vi "Rename LVClass_rcf.vi"(7 "App reference":refnum<vi>, 8 "error in (no error)":errorcluster, 10 "New Class Name":string, 11 "LVClass Path":path) -> (0 "error out":errorcluster, 3 "Updated LVClass Path":path)   [LabVIEW 2009]
uses:
  <userlib>/_OpenG.lib/file/file.llb/Strip Path Extension - String__ogtk.vi
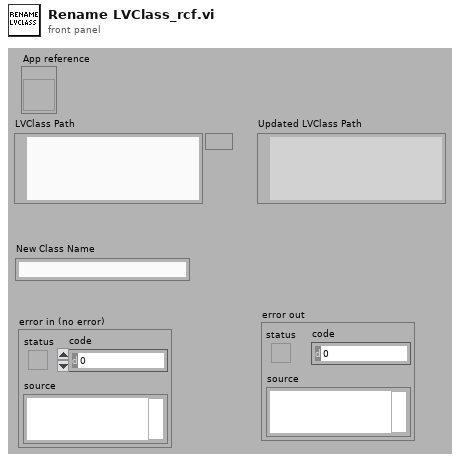
[diagram p1: front panel]
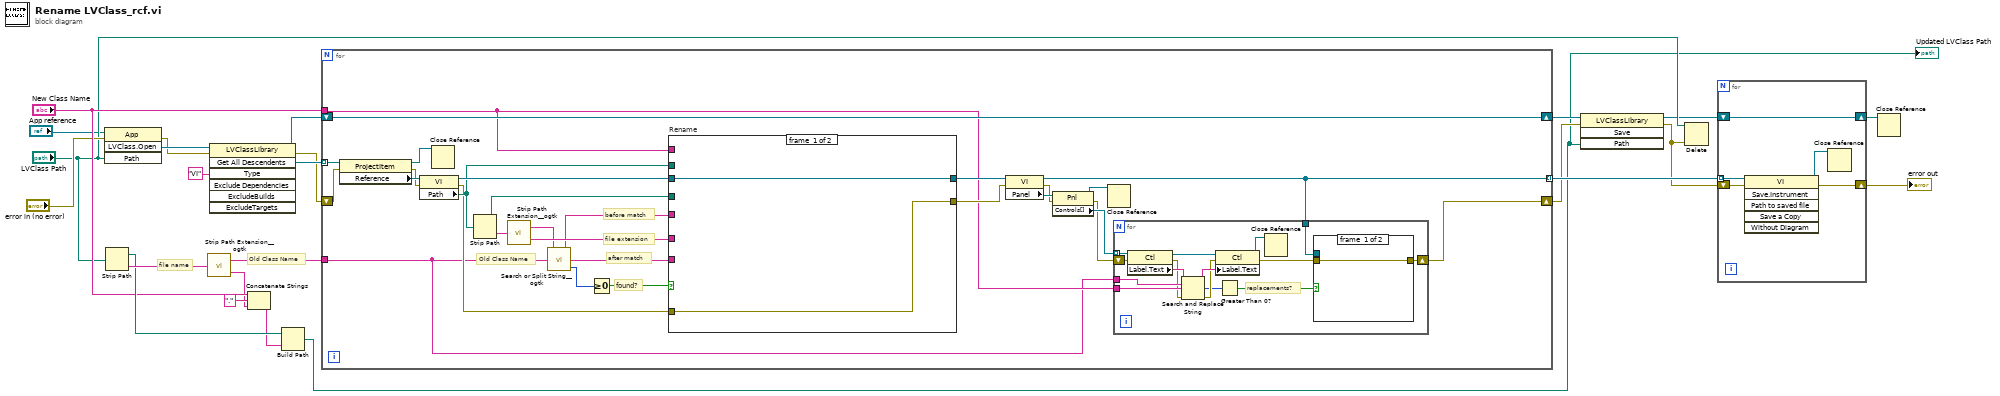
[diagram p0: block diagram]
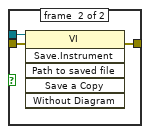
[diagram p2: hidden frame]
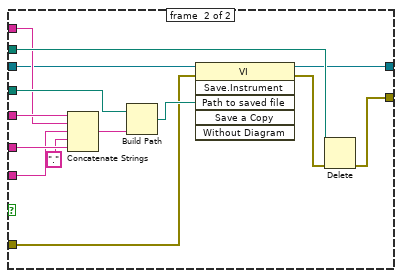
[diagram p3: hidden frame]
diagram:
  # "file name"
  # "Old Class Name"
  n1 = invoke class="App" method="LVClass.Open"(reference="App reference", error in="error in (no error)", "Path"="LVClass Path") -> (error out=w3:errorcluster, "LVClass.Open"=w4:refnum<vi>)  [unwired: 1 in, 2 out]
  n2 = Strip Path(path="LVClass Path") -> (stripped path=w18:path, name=w21:string)
  n3 = call-poly <userlib>:"Strip Path Extension__ogtk.vi"("path"=w21) -> ("root"=w22:string, "extension"=w15:string)
  n4 = invoke class="LVClassLibrary" method="Get All Descendents"(reference=w4, error in=w3, "Type"="VI") -> (reference out=w20:refnum<vi>, error out=w11:errorcluster, "All Descendents"=w23:refnum<vi>[])  [unwired: 4 in, 4 out]
  n5 = Concatenate Strings("New Class Name", "." ("string"), w15) -> (w14:string)
  n6 = Build Path(base path=w18, name or relative path=w14) -> (appended path=w2:path)
  "Updated LVClass Path" <- w2
  n7 = for {
    tunnel: w23 -> [w52] mode=indexing
    tunnel: "New Class Name" -> [w28]
    tunnel: w22 -> [w27]
    shift-right: [w40] -> w19
    shift-left: w20 -> [w40]
    tunnel: [w26] -> w13 mode=indexing
    shift-right: [w25] -> w12
    shift-left: w11 -> [w39]
    # "file extension"
    # "before match"
    # "after match"
    # "found?"
    # "Old Class Name"
    n8 = property class="ProjectItem"(reference=w52, error in=w39) -> (reference out=w36:refnum<vi>, error out=w38:errorcluster, "Reference"=w51:refnum<vi>)
    n9 = property class="VI"(reference=w51, error in=w38) -> (reference out=w49:refnum<vi>, error out=w37:errorcluster, "Path"=w47:path)
    n10 = Close Reference(reference=w36) -> ()  [unwired: 1 in, 1 out]
    n11 = Strip Path(path=w47) -> (stripped path=w48:path, name=w50:string)
    n12 = call-poly <userlib>:"Strip Path Extension__ogtk.vi"("path"=w50) -> ("root"=w45:string, "extension"=w46:string)
    n13 = call <userlib>:"Search or Split String__ogtk.vi"("search string/char (-)"=w27, "string"=w45) -> ("offset after match"=w44:i32, "substring after match"=w41:string, "substring before match"=w42:string)  [unwired: 1 in]
    n14 = Greater Or Equal To 0?(x=w44) -> (x >= 0?=w43:bool)
    n15 = case "Rename" shown="True" w43 {
      tunnel: w49 -> [w73 w74]
      tunnel: w46 -> [_ w87]
      tunnel: w48 -> [_ w85]
      tunnel: w47 -> [_ w81]
      tunnel: w42 -> [_ w80]
      tunnel: w28 -> [_ w76]
      tunnel: w41 -> [_ w79]
      tunnel: [w73 w78] -> w30
      tunnel: [w72 w77] -> w29
      tunnel: w37 -> [w72 w75]
      frame #0 {
      }
      frame #1 {
        n16 = Concatenate Strings(w80, w76, w79, "." ("string"), w87) -> (w84:string)
        n17 = Build Path(base path=w85, name or relative path=w84) -> (appended path=w83:path)
        n18 = invoke class="VI" method="Save.Instrument"(reference=w74, error in=w75, "Path to saved file"=w83) -> (reference out=w78:refnum<vi>, error out=w82:errorcluster)  [unwired: 3 in, 4 out]
        n19 = Delete(path (use dialog)=w81, error in=w82) -> (error out=w77:errorcluster)  [unwired: 3 in, 2 out]
      }
    }
    n20 = property class="VI"(reference=w30, error in=w29) -> (reference out=w26:refnum<vi>, error out=w32:errorcluster, "Panel"=w35:refnum<vi>)
    n21 = property class="Pnl"(reference=w35, error in=w32) -> (reference out=w31:refnum<vi>, error out=w33:errorcluster, "Controls[]"=w34:refnum<vi>[])
    n22 = Close Reference(reference=w31) -> ()  [unwired: 1 in, 1 out]
    n23 = for {
      tunnel: w34 -> [w67] mode=indexing
      tunnel: w27 -> [w64]
      tunnel: w28 -> [w63]
      shift-right: [w57] -> w25
      shift-left: w33 -> [w59]
      tunnel: w26 -> [w56]
      # "replacements?"
      n24 = property class="Ctl"(reference=w67, error in=w59) -> (reference out=w66:refnum<vi>, error out=w61:errorcluster, "Label.Text"=w65:string)
      n25 = Search and Replace String(input string=w65, search string=w64, replace string=w63, error in=w61) -> (result string=w62:string, number of replacements=w54:i32, error out=w60:errorcluster)  [unwired: 4 in, 1 out]
      n26 = property class="Ctl"(reference=w66, error in=w60, "Label.Text"=w62) -> (reference out=w58:refnum<vi>, error out=w55:errorcluster)
      n27 = Greater Than 0?(x=w54) -> (x > 0?=w53:bool)
      n28 = Close Reference(reference=w58) -> ()  [unwired: 1 in, 1 out]
      n29 = case shown="True" w53 {
        tunnel: [w68 w71] -> w57
        tunnel: w56 -> [_ w70]
        tunnel: w55 -> [w68 w69]
        frame #0 {
        }
        frame #1 {
          n30 = invoke class="VI" method="Save.Instrument"(reference=w70, error in=w69) -> (error out=w71:errorcluster)  [unwired: 4 in, 5 out]
        }
      }
    }
  }
  n31 = invoke class="LVClassLibrary" method="Save"(reference=w19, error in=w12, "Path"=w2) -> (reference out=w6:refnum<vi>, error out=w8:errorcluster)  [unwired: 1 in, 2 out]
  n32 = Delete(path (use dialog)="LVClass Path", error in=w8) -> ()  [unwired: 3 in, 3 out]
  n33 = for {
    tunnel: w13 -> [w92] mode=indexing
    shift-right: [w90] -> w9
    shift-left: w8 -> [w91]
    shift-right: [w88] -> w5
    shift-left: w6 -> [w88]
    n34 = invoke class="VI" method="Save.Instrument"(reference=w92, error in=w91) -> (reference out=w89:refnum<vi>, error out=w90:errorcluster)  [unwired: 4 in, 4 out]
    n35 = Close Reference(reference=w89) -> ()  [unwired: 1 in, 1 out]
  }
  "error out" <- w9
  n36 = Close Reference(reference=w5) -> ()  [unwired: 1 in, 1 out]
